vi "CmdMono.vi"(4 "Busy":refnum<vi>, 5 "Valid Read Time Out (60 sec)":dbl=60.0, 6 "Scan Speed (nm/min)":dbl=100.0 min=1.0 max=500.0, 7 "Write Wait (10 ms)":u32=10, 8 "error in (no error)":errorcluster, 9 "Wavelength (nm)":dbl=100.0 min=0.0 max=2000.0, 10 "Cmd":u16(ring) items=["nm", "goto", "nm/min", "VIS grating", "IR grating"], 11 "Mono Port":refnum<visa-resource-name>="COM5") -> (0 "error out":errorcluster, 1 "Read Error":bool, 2 "Response":string, 3 "Mono Port Out":refnum<visa-resource-name>)   [LabVIEW 2013]
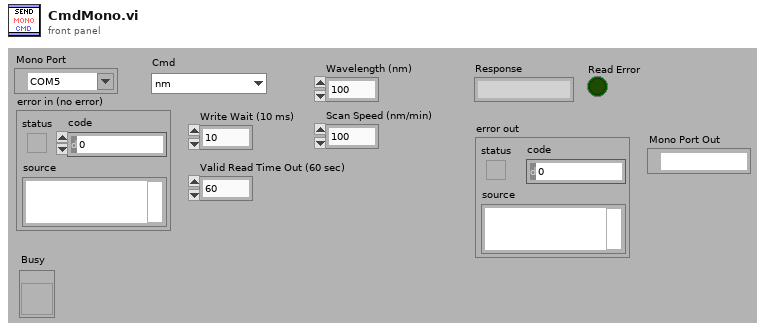
[diagram p1: front panel]
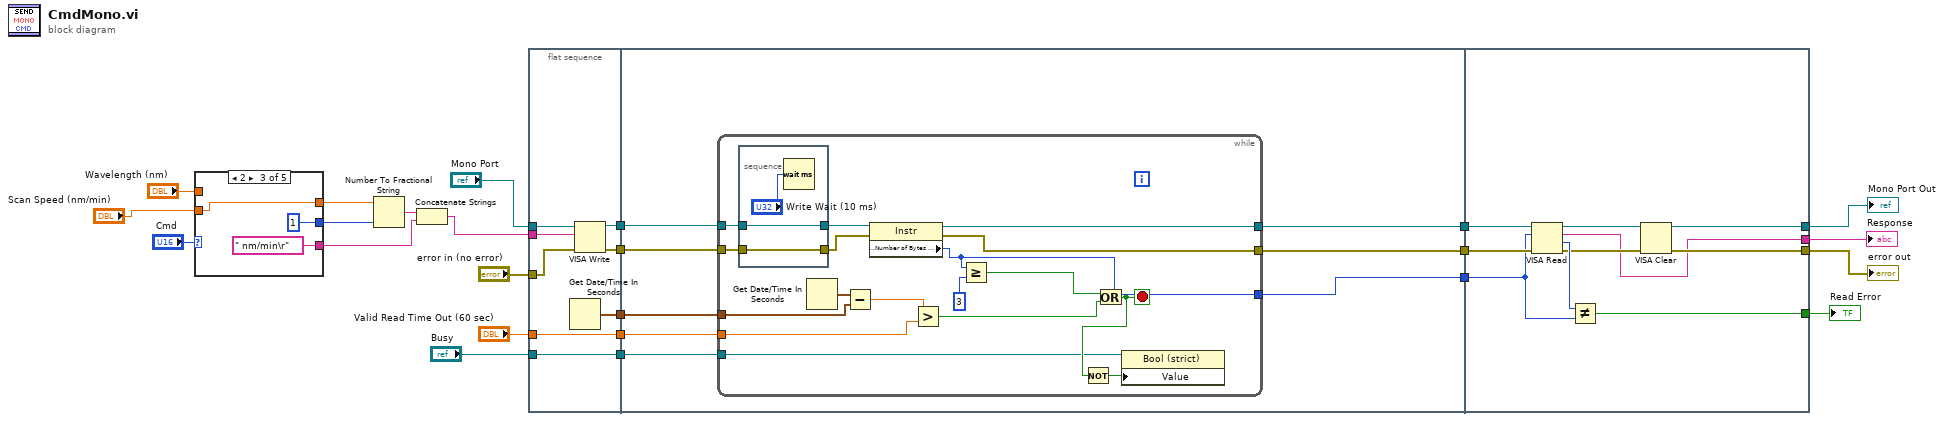
[diagram p0: block diagram]
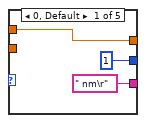
[diagram p2: hidden frame]
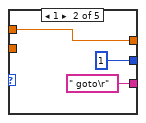
[diagram p3: hidden frame]
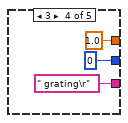
[diagram p4: hidden frame]
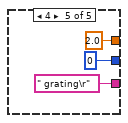
[diagram p5: hidden frame]
diagram:
  n1 = case shown="2" "Cmd" {
    tunnel: [" nm\r" " goto\r" " nm/min\r" " grating\r" " grating\r"] -> w23
    tunnel: [i16 1 ("precision (6)") i16 1 ("precision (6)") i16 1 ("precision (6)") i16 0 ("precision (6)") i16 0 ("precision (6)")] -> w21
    tunnel: "Wavelength (nm)" -> [w25 w28 _ _ _]
    tunnel: [w25 w28 w31 1.0 ("Cmd Value") 2.0 ("Cmd Value")] -> w19
    tunnel: "Scan Speed (nm/min)" -> [_ _ w31 _ _]
    frame 0, Default {
    }
    frame 1 {
    }
    frame 2 {
    }
    frame 3 {
    }
    frame 4 {
    }
  }
  n2 = Number To Fractional String(number=w19, precision (6)=w21) -> (F-format string=w22:string)  [unwired: 2 in]
  n3 = Concatenate Strings(w22, w23) -> (w8:string)
  n4 = flat-sequence {
    tunnel: "Mono Port" -> [w47]
    tunnel: "error in (no error)" -> [w46]
    tunnel: w8 -> [w45]
    tunnel: [w44] -> w18
    tunnel: [w43] -> w17
    tunnel: [w42] -> w16
    tunnel: "Valid Read Time Out (60 sec)" -> [w41]
    tunnel: [w41] -> w15
    tunnel: [w40] -> w2
    tunnel: "Busy" -> [w40]
    tunnel: w18 -> [w55]
    tunnel: w17 -> [w54]
    tunnel: w16 -> [w53]
    tunnel: [w52] -> w14
    tunnel: [w51] -> w13
    tunnel: [w50] -> w12
    tunnel: w15 -> [w49]
    tunnel: w2 -> [w48]
    tunnel: w14 -> [w85]
    tunnel: w13 -> [w84]
    tunnel: [w78] -> w5
    tunnel: [w77] -> w4
    tunnel: [w76] -> w6
    tunnel: [w82] -> w3
    tunnel: w12 -> [w81]
    frame #0 {
      n5 = Get Date/Time In Seconds() -> (seconds since 1Jan1904=w44:timestamp)
      n6 = VISA Write(VISA resource name=w47, write buffer=w45, error in (no error)=w46) -> (VISA resource name out=w43:refnum<visa-resource-name>, error out=w42:errorcluster)  [unwired: 1 out]
    }
    frame #1 {
      n7 = while {
        tunnel: w55 -> [w70]
        tunnel: w54 -> [w67]
        tunnel: w53 -> [w68]
        tunnel: [w64] -> w52
        tunnel: [w63] -> w51
        tunnel: [w61] -> w50
        tunnel: w49 -> [w62]
        tunnel: w48 -> [w57]
        stop <- w58 stop-if-true
        n8 = stacked-sequence {
          tunnel: [w74] -> w65
          tunnel: w67 -> [w75]
          tunnel: [w75] -> w66
          tunnel: w68 -> [w74]
          frame #0 {
            n9 = Wait (ms)(milliseconds to wait="Write Wait (10 ms)") -> ()  [unwired: 1 out]
          }
        }
        n10 = Get Date/Time In Seconds() -> (seconds since 1Jan1904=w72:timestamp)
        n11 = Subtract(x=w72, y=w70) -> (x-y=w71:dbl)
        n12 = property class="Instr"(reference=w66, error in=w65) -> (reference out=w64:refnum<visa-resource-name>, error out=w63:errorcluster, "Serial Settings:Number of Bytes at Serial Port"=w61:u32)
        n13 = Greater?(x=w71, y=w62) -> (0:w69:bool)
        n14 = Greater Or Equal?(x=w61, y=u32 3) -> (x >= y?=w59:bool)
        n15 = Or(x=w59, y=w69) -> (x .or. y?=w58:bool)
        n16 = Not(x=w58) -> (.not. x?=w56:bool)
        n17 = property class="Bool (strict)"(reference=w57, "Value"=w56) -> ()  [unwired: 1 in, 2 out]
      }
    }
    frame #2 {
      n18 = VISA Read(VISA resource name=w85, byte count=w81, error in (no error)=w84) -> (VISA resource name out=w80:refnum<visa-resource-name>, read buffer=w76:string, return count=w83:u32, error out=w79:errorcluster)
      n19 = Not Equal?(x=w83, y=w81) -> (x != y?=w82:bool)
      n20 = VISA Clear(VISA resource name=w80, error in (no error)=w79) -> (VISA resource name out=w78:refnum<visa-resource-name>, error out=w77:errorcluster)
    }
  }
  "Read Error" <- w3
  "error out" <- w4
  "Response" <- w6
  "Mono Port Out" <- w5
